vi "FTW-Ether-Destroy.vi"(5 "Force Destroy?":bool, 11 "error in":errorcluster) -> (15 "error out":errorcluster)   [LabVIEW 2012, in "FTW-Actor.lvlib" / "FTW-Ether.lvclass"]
uses:
  FTW-Ether.lvclass
  EventLogger/FTW-Logger.lvclass
  FTW-Ether-Instance.vi
  ZMQ/FTW-Endpoint-ZMQ.lvclass
panel:
  # "Inputs"
  # "Outputs"
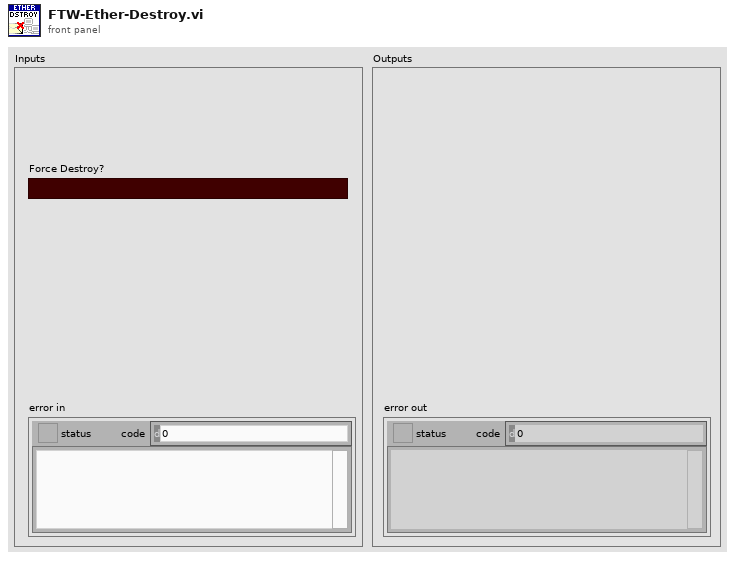
[diagram p1: front panel]
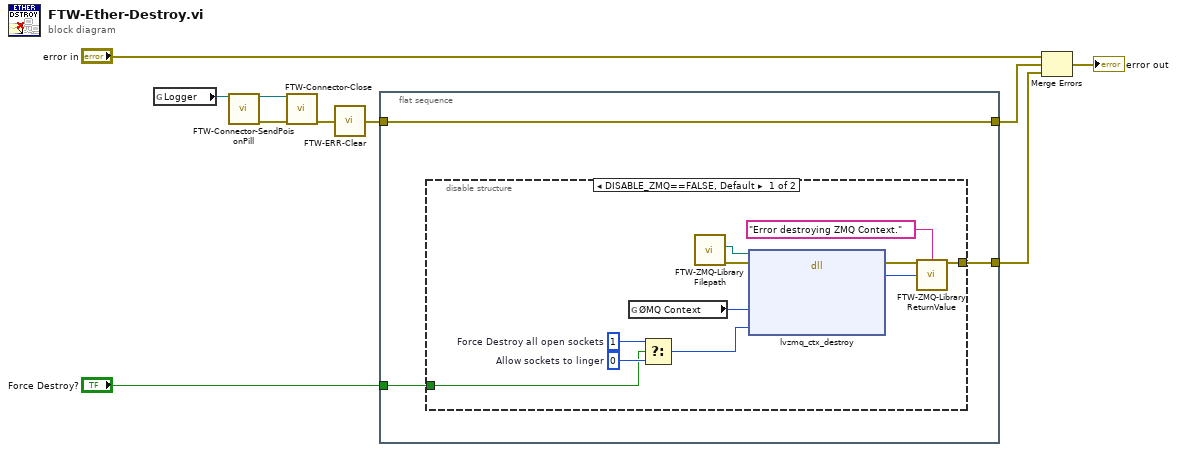
[diagram p0: block diagram]
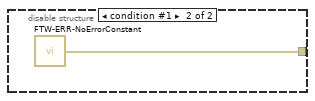
[diagram p2: hidden frame]
diagram:
  n1 = global read "FTW-Ether-Instance.vi" "Logger"() -> (w1:refnum<class "FTW-Logger.lvclass">)
  n2 = call-dynamic "FTW-Connector-SendPoisonPill.vi"("Actor Reference"=w1) -> ("Actor Reference out"=w8:refnum<class "FTW-Logger.lvclass">, "error out"=w7:errorcluster)  [unwired: 13 in]
  n3 = call-dynamic "FTW-Connector-Close.vi"("FTW Actor Reference"=w8, "error in"=w7) -> ("error out"=w3:errorcluster)  [unwired: 13 in]
  n4 = call "FTW-ERR-Clear.vi"("error to snuff"=w3) -> ("no error"=w2:errorcluster)
  n5 = flat-sequence {
    tunnel: "Force Destroy?" -> [w13]
    tunnel: w2 -> [w12]
    tunnel: [w12] -> w5
    tunnel: [w11] -> w4
    frame #0 {
      n6 = disable-structure shown="DISABLE_ZMQ==FALSE, Default" {
        disable-tunnel: w13 -> [w16 _]
        disable-tunnel: [w15 w25] -> w11
        frame condition #0 (active) {
          w24 = 1  # Force Destroy all open sockets
          w22 = 0  # Allow sockets to linger
          n7 = global read "FTW-Ether-Instance.vi" "ØMQ Context"() -> (w14:u64)
          n8 = Select(t=w24, s=w16, f=w22) -> (s? t:f=w23:i32)
          n9 = call "FTW-ZMQ-LibraryFilepath.vi"() -> ("error out"=w18:errorcluster, "FTW-ZMQ Library Filepath"=w19:path)  [unwired: 9 in, 1 out]
          n10 = dll-call lib="?" fn="lvzmq_ctx_destroy" ("zmq_labview.dll:lvzmq_term")(path in=w19, error in=w18, "Context"=w14, "Flags"=w23) -> (error out=w21:errorcluster, "Return Value"=w20:i32)  [unwired: 5 in, 1 out]
          n11 = call "FTW-ZMQ-LibraryReturnValue.vi"("error in"=w21, "Error Message"="Error destroying ZMQ Context.", "Return Value"=w20) -> ("error out"=w15:errorcluster)  [unwired: 12 in]
        }
        frame condition #1 {
          n12 = call "FTW-ERR-NoErrorConstant.vi"() -> ("no error"=w25:errorcluster)
        }
      }
    }
  }
  n13 = Merge Errors("error in", w5, w4) -> (→"error out":errorcluster)
